vi "SPCM_simple_measure.vi"(2 "Clear memory":bool=TRUE, 3 "Collection Time":sgl=3.0 format="%.4f", 4 "Meas page":u16) -> (0 "SPC error":T3={"Error code"=0, "Message"="No errors"}, 1 "Waveform Graph":u16[][](graph))   [LabVIEW 2011]
uses:
  Program Files (x86)/BH/SPCM/DLL/spcm_functions_lv10.llb/error.ctl
  Program Files (x86)/BH/SPCM/DLL/spcm_functions_lv10.llb/Global_SPCM_vars.vi
  SPCM_DLL_path.vi
panel:
  in  "Active module":u16(ring) items=["Module 0", "Module 1", "Module 2", "Module 3", "Module 4", "Module 5", "Module 6", "Module 7"]
  out "Modules in use":T1
  in  "No of routing bits":u16 max=14 step=1
  in  "ADC resolution":u16=10 min=6 max=12 step=2
  out "SPC_rates":T2 {"Adc_rate" format="%.2e"; "Tac_rate" format="%.2e"; "Cfd_rate" format="%.2e"; "Sync_rate" format="%.2e"}
  in  "Current Collection Time":sgl=3.0 format="%.4f"
  in  "Current page":u16
  out "Output Array":u16[][](array[numeric])
  in  "Repeat Measurement":bool
  out "SYNC LED":bool=TRUE
  out "state value":i16 format="%.0x"
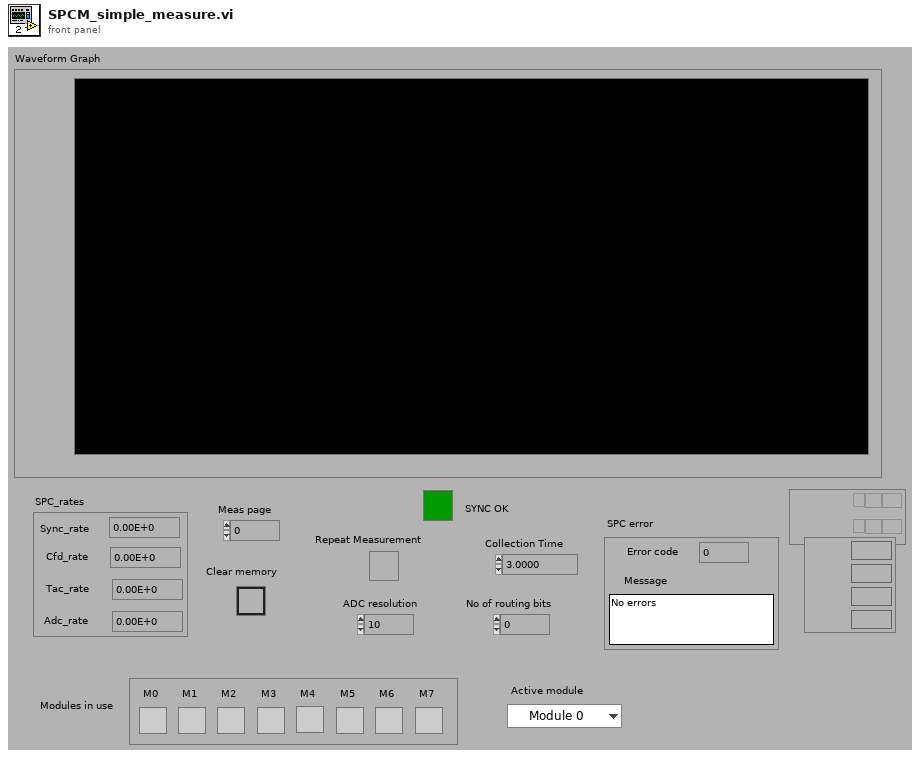
[diagram p1: front panel]
types:
  T1 = cluster{"M0":bool, "M1":bool, "M2":bool, "M3":bool, "M4":bool, "M5":bool, "M6":bool, "M7":bool}
  T2 = cluster{"Sync_rate":sgl, "Cfd_rate":sgl, "Tac_rate":sgl, "Adc_rate":sgl}
  T3 = typedef "error.ctl" = cluster{"Error code":i16, "Message":string}
  T4 = typedef "SPCdata.ctl" = cluster{"Base Address":u16, "Init status":i16, "CFD Limit Low [mV]":sgl, "CFD Limit High [mV]":sgl, "CFD ZC Level [mV]":sgl, "CFD Holdoff [ns]":sgl, "SYNC ZC Level [mV]":sgl, "SYNC Holdoff [ns]":sgl, "SYNC Threshold [mV]":sgl, "TAC Range [ns]":sgl, "SYNC Freq Divider":i16, "TAC Gain":i16, "TAC Offset [%]":sgl, "TAC Limit Low [%]":sgl, "TAC Limit High [%]":sgl, "ADC Resolution":i16, "Ext Latch Delay":i16, "Collection Time [s]":sgl, "Display Time [s]":sgl, "Repeat Time [s]":sgl, "Stop on Time":i16, "Stop on Overflow":i16, "Dither Range":i16, "Count Increment":i16, "Memory Bank":i16, "Dead Time Compensation":i16, "Scan Control":u16, "Routing Mode":i16, "TAC Enable Hold":sgl, "Slot No of PCI Module":i16, "Operation Mode":u16, "Scan Size X":u32, "Scan Size Y":u32, "Scan Routing Size X ":u32, "Scan Routing Size Y":u32, "Scan Flyback":u32, "Scan Borders":u32, "Scan Polarity":u16, "Pixel Clock Source":u16, "Line Compression":u16, "External Trigger Condition":u16, "Pixel Time [s]":sgl, "External pixel clock divider":u32, "Rate Counting Time":sgl, "Macro Time Clock  ":i16, "ADD Signal Source":i16, "Test EEPROM":i16, "ADC Zoom":i16, "Image Size X":u32, "Image Size Y":u32, "Image Routing Size X":u32, "Image Routing Size Y":u32, "XY Gain":i16, "Master Clock":i16, "ADC Sample Delay":i16, "Detector Type":i16, "X Axis Type":i16, "Channel enable ( DPC-230)":u32, "Channel slope ( DPC-230)":u32, "Channel spec_no ( DPC-230)":u32}
  T5 = typedef "mem_config.ctl" = cluster{"max_block_no":i32, "blocks_per_frame":i32, "frames_per_page":i32, "maxpage":i32, "block_length":i16}
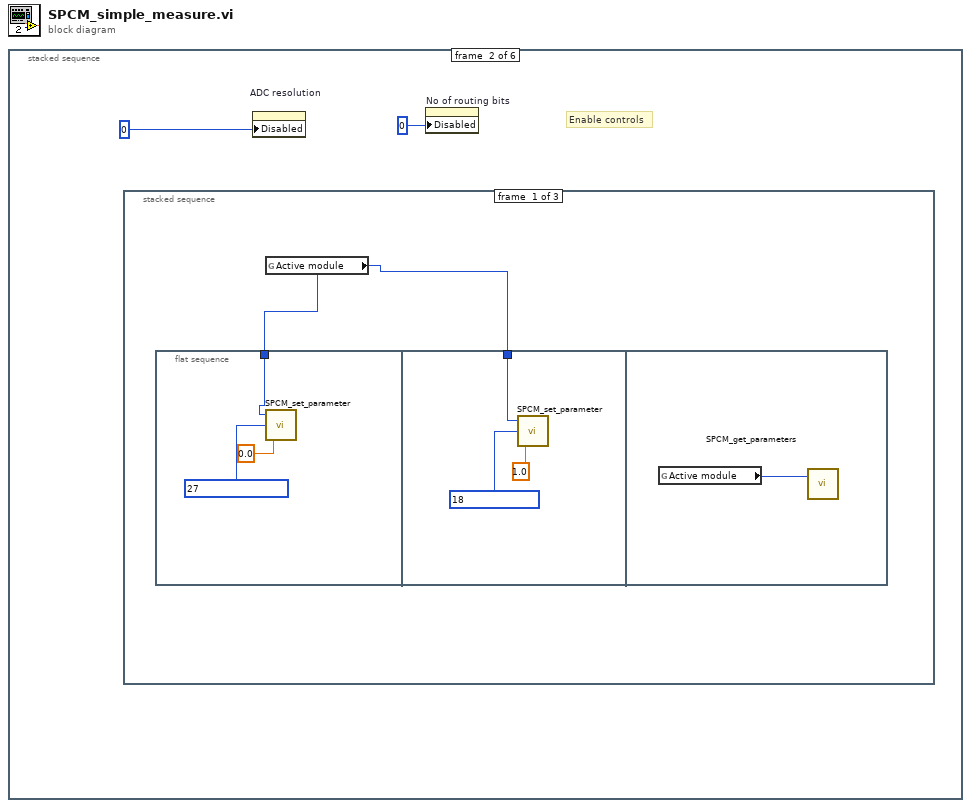
[diagram p0: block diagram]
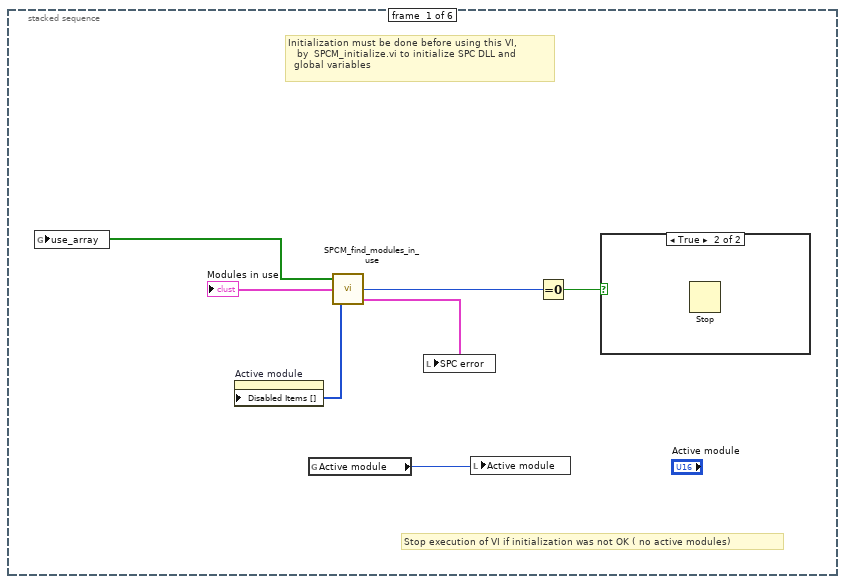
[diagram p2: hidden frame]
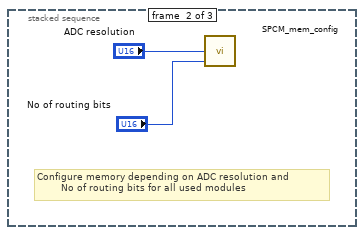
[diagram p4: hidden frame]
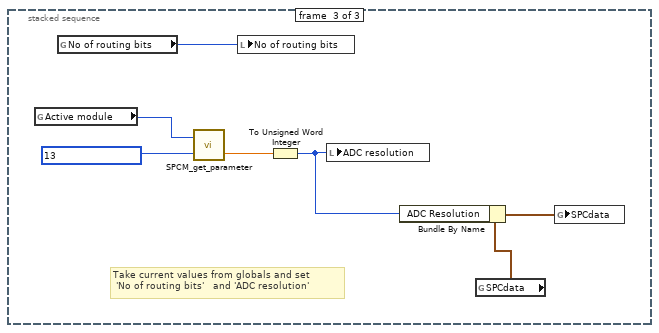
[diagram p5: hidden frame]
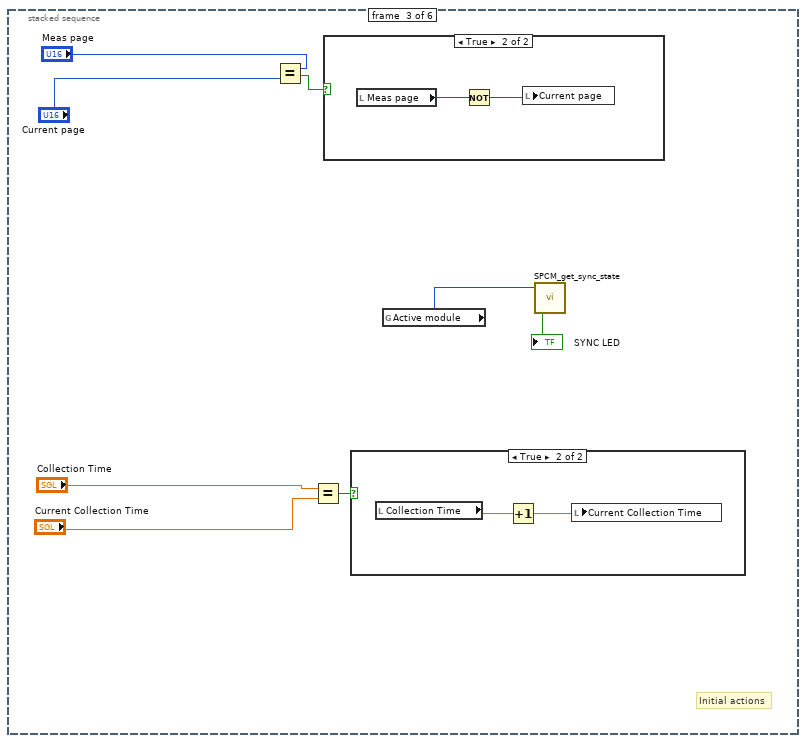
[diagram p6: hidden frame]
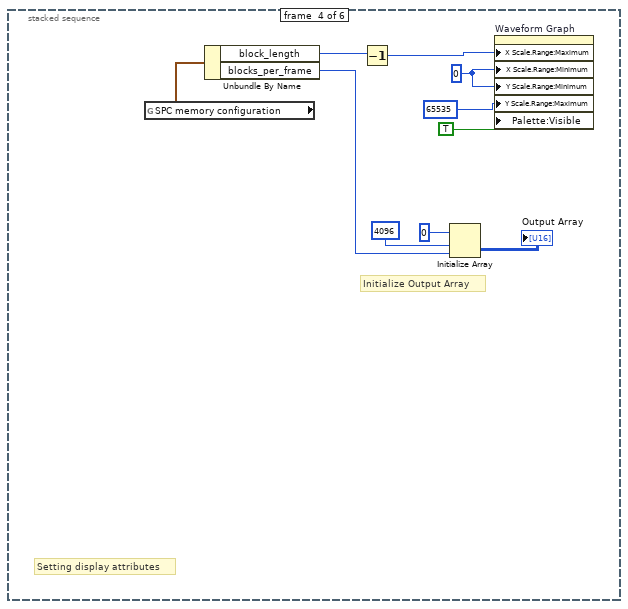
[diagram p9: hidden frame]
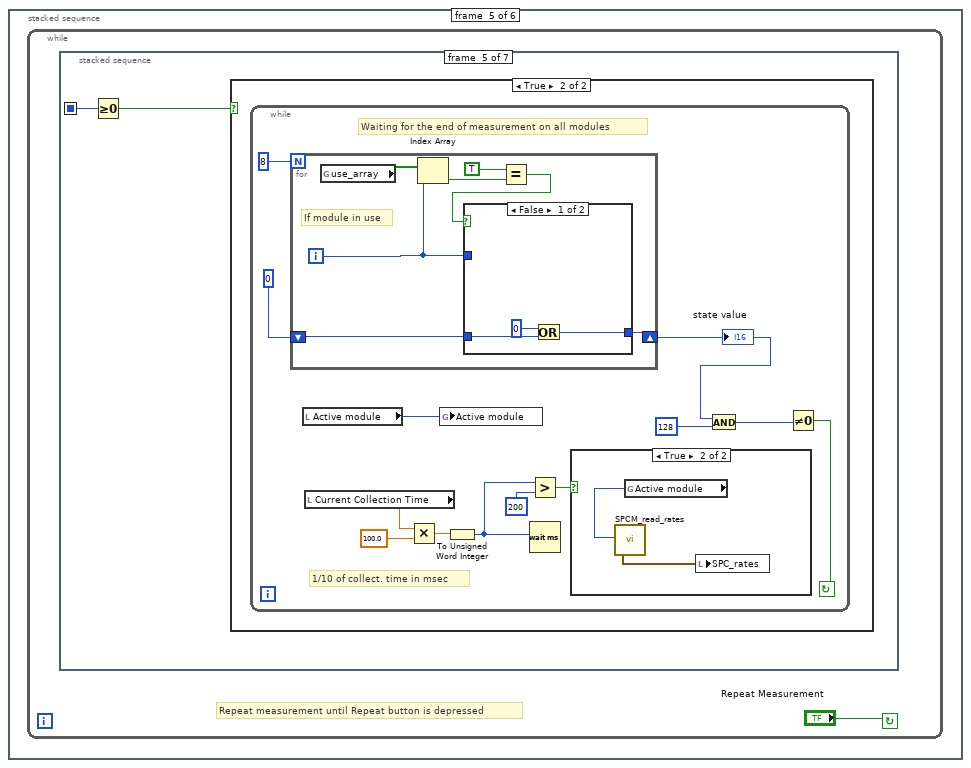
[diagram p10: hidden frame]
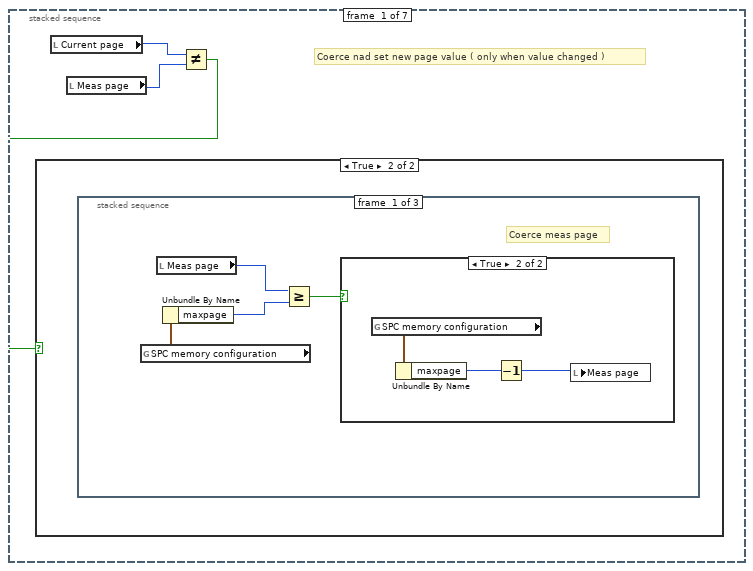
[diagram p11: hidden frame]
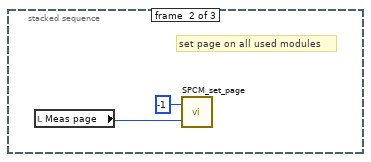
[diagram p14: hidden frame]
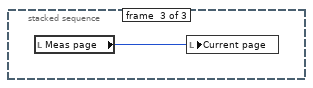
[diagram p15: hidden frame]
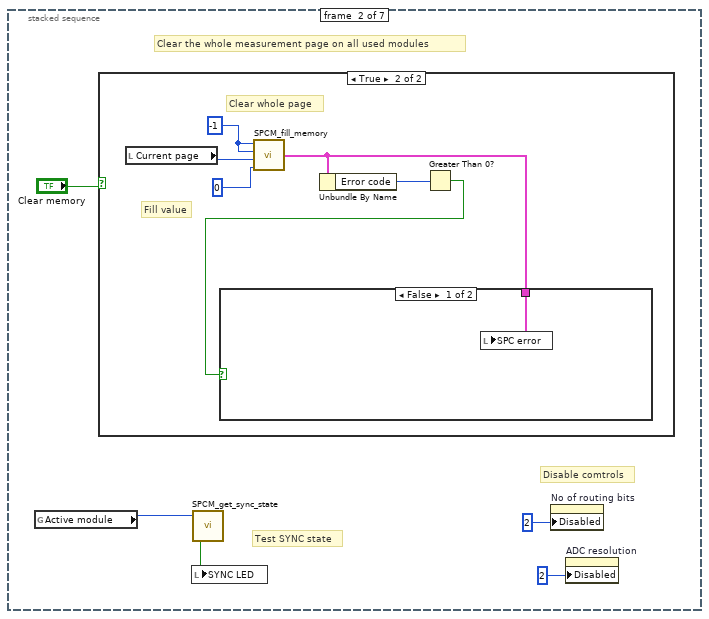
[diagram p16: hidden frame]
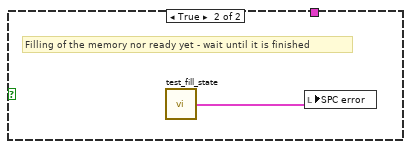
[diagram p18: hidden frame]
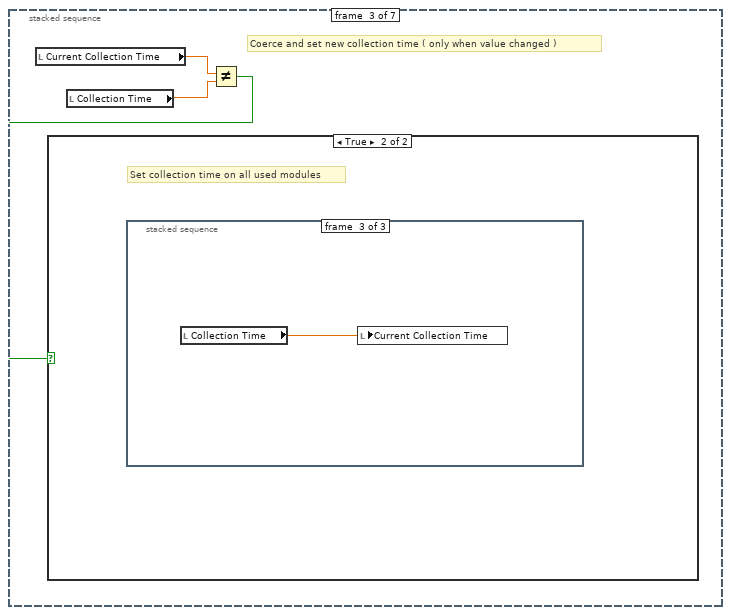
[diagram p19: hidden frame]
diagram:
  n1 = stacked-sequence {
    frame #0 {
      # "Stop execution of VI if initialization was not OK ( no active modules)"
      # "Initialization must be done before using this VI, \n   by  SPCM_initialize.vi to initialize SPC DLL and \n  global variables"
      n2 = global read "Global_SPCM_vars.vi" "Active module"() -> (w2:i16)
      n3 = call "SPCM_find_modules_in_use.vi"() -> ("SPC error"=w6:T3, "Number of used modules"=w4:i16, "Disabled Items"=w3:i32[], "Use LEDs"=→"Modules in use":T1, "use_array"=w1:bool[])  [unwired: 1 out]
      n4 = global write "Global_SPCM_vars.vi" "use_array"(w1) -> ()
      n5 = property on="Active module" class="Ring (strict)"("Disabled Items []"=w3) -> ()  [unwired: 2 in, 2 out]
      n6 = local write "SPC error"(w6) -> ()
      n7 = local write "Active module"(w2) -> ()
      n8 = Equal To 0?(x=w4) -> (x = 0?=w5:bool)
      n9 = case shown="True" w5 {
        frame False {
        }
        frame True {
          n10 = Stop() -> ()  [unwired: 1 in]
        }
      }
    }
    frame #1 {
      # "Enable controls"
      n11 = stacked-sequence {
        frame #0 {
          n12 = flat-sequence {
            tunnel: w10 -> [w11]
            tunnel: w10 -> [w14]
            frame #0 {
              n13 = call "SPCM_set_parameter.vi"("Parameter Value"=sgl 0.0, "SPC parameter ID"=u16 27, "Module no"=w11) -> ()  [unwired: 1 out]
            }
            frame #1 {
              n14 = call "SPCM_set_parameter.vi"("Parameter Value"=sgl 1.0, "SPC parameter ID"=u16 18, "Module no"=w14) -> ()  [unwired: 1 out]
            }
            frame #2 {
              n15 = global read "Global_SPCM_vars.vi" "Active module"() -> (w17:i16)
              n16 = call "SPCM_get_parameters.vi"("Module no"=w17) -> ()  [unwired: 2 out]
            }
          }
          n17 = global read "Global_SPCM_vars.vi" "Active module"() -> (w10:i16)
        }
        frame #1 {
          # "Configure memory depending on ADC resolution and\n        No of routing bits for all used modules"
          n18 = call "SPCM_mem_config.vi"("No of routing bits"="No of routing bits", "ADC resolution"="ADC resolution") -> ()  [unwired: 1 in, 2 out]
        }
        frame #2 {
          # "Take current values from globals and set\n 'No of routing bits'   and 'ADC resolution'"
          n19 = global read "Global_SPCM_vars.vi" "Active module"() -> (w23:i16)
          n20 = global read "Global_SPCM_vars.vi" "No of routing bits"() -> (w24:u16)
          n21 = call "SPCM_get_parameter.vi"("SPC parameter ID"=u16 13, "Module no"=w23) -> ("Current Parameter Value"=w26:sgl)  [unwired: 1 out]
          n22 = local write "No of routing bits"(w24) -> ()
          n23 = To Unsigned Word Integer(number=w26) -> (unsigned 16bit integer=w25:u16)
          n24 = local write "ADC resolution"(w25) -> ()
          n25 = global read "Global_SPCM_vars.vi" "SPCdata"() -> (w21:T4)
          n26 = Bundle By Name(cluster=w21, "ADC Resolution"=w25) -> (w22:T4)
          n27 = global write "Global_SPCM_vars.vi" "SPCdata"(w22) -> ()
        }
      }
      n28 = property on="ADC resolution" class="DigNum (strict)"("Disabled"=u8 0 ("Write Attribute")) -> ()  [unwired: 2 in, 2 out]
      n29 = property on="No of routing bits" class="DigNum (strict)"("Disabled"=u8 0 ("Write Attribute")) -> ()  [unwired: 2 in, 2 out]
    }
    frame #2 {
      # "Initial actions"
      n30 = Equal?(x="Meas page", y="Current page") -> (x = y?=w31:bool)
      n31 = Equal?(x="Collection Time", y="Current Collection Time") -> (x = y?=w28:bool)
      n32 = case shown="True" w31 {
        frame False {
        }
        frame True {
          n33 = local read "Meas page"() -> (w38:u16)
          n34 = Not(x=w38) -> (.not. x?=w37:u16)
          n35 = local write "Current page"(w37) -> ()
        }
      }
      n36 = case shown="True" w28 {
        frame False {
        }
        frame True {
          n37 = local read "Collection Time"() -> (w36:sgl)
          n38 = Increment(x=w36) -> (x+1=w35:sgl)
          n39 = local write "Current Collection Time"(w35) -> ()
        }
      }
      n40 = global read "Global_SPCM_vars.vi" "Active module"() -> (w27:i16)
      n41 = call "SPCM_get_sync_state.vi"("Module no"=w27) -> ("LED"=→"SYNC LED":bool)  [unwired: 2 out]
    }
    frame #3 {
      w43 = u16 0 ("Write Attribute")
      # "Initialize Output Array"
      # "Setting display attributes"
      n42 = global read "Global_SPCM_vars.vi" "SPC memory configuration"() -> (w48:T5)
      n43 = Unbundle By Name(w48) -> ("block_length"=w40:i16, "blocks_per_frame"=w44:i32)
      n44 = Decrement(x=w40) -> (x-1=w47:i16)
      n45 = Initialize Array(u16 0 ("Element Data"), 4096 ("Dimension Size"), w44) -> (→"Output Array":u16[][])
      n46 = property on="Waveform Graph" class="WFGraph (strict)"("X Scale.Range:Maximum"=w47, "X Scale.Range:Minimum"=w43, "Y Scale.Range:Minimum"=w43, "Y Scale.Range:Maximum"=u16 65535 ("Write Attribute"), "Palette:Visible"=TRUE ("Write Attribute")) -> ()  [unwired: 2 in, 2 out]
    }
    frame #4 {
      n47 = while {
        stop <- "Repeat Measurement" continue-if-true
        # "Repeat measurement until Repeat button is depressed"
        n48 = stacked-sequence {
          seq-local: [_ _ _ w88 _ _ _] -> [_ _ _ _ w104 w135 _]
          frame #0 {
            # "Coerce nad set new page value ( only when value changed )"
            n49 = local read "Current page"() -> (w52:u16)
            n50 = local read "Meas page"() -> (w50:u16)
            n51 = Not Equal?(x=w52, y=w50) -> (x != y?=w51:bool)
            n52 = case shown="True" w51 {
              frame False {
              }
              frame True {
                n53 = stacked-sequence {
                  frame #0 {
                    # "Coerce meas page"
                    n54 = global read "Global_SPCM_vars.vi" "SPC memory configuration"() -> (w56:T5)
                    n55 = local read "Meas page"() -> (w53:u16)
                    n56 = Unbundle By Name(w56) -> ("maxpage"=w55:i32)
                    n57 = Greater Or Equal?(x=w53, y=w55) -> (x >= y?=w54:bool)
                    n58 = case shown="True" w54 {
                      frame False {
                      }
                      frame True {
                        n59 = global read "Global_SPCM_vars.vi" "SPC memory configuration"() -> (w59:T5)
                        n60 = Unbundle By Name(w59) -> ("maxpage"=w58:i32)
                        n61 = Decrement(x=w58) -> (x-1=w57:i32)
                        n62 = local write "Meas page"(w57) -> ()
                      }
                    }
                  }
                  frame #1 {
                    # "set page on all used modules"
                    n63 = local read "Meas page"() -> (w61:u16)
                    n64 = call "SPCM_set_page.vi"("Page"=w61, "Module no"=i16 -1) -> ()  [unwired: 1 out]
                  }
                  frame #2 {
                    n65 = local read "Meas page"() -> (w62:u16)
                    n66 = local write "Current page"(w62) -> ()
                  }
                }
              }
            }
          }
          frame #1 {
            # "Disable comtrols"
            # "Test SYNC state"
            # "Clear the whole measurement page on all used modules"
            n67 = global read "Global_SPCM_vars.vi" "Active module"() -> (w65:i16)
            n68 = case shown="True" "Clear memory" {
              frame False {
              }
              frame True {
                w71 = i16 -1 ("Block")
                # "Clear whole page"
                # "Fill value"
                n69 = local read "Current page"() -> (w72:u16)
                n70 = call "SPCM_fill_memory.vi"("Fill value"=u16 0, "Page"=w72, "Block"=w71, "Module no"=w71) -> ("SPC error"=w68:cluster{"Error code":i16, "Message":string})
                n71 = Unbundle By Name(w68) -> ("Error code"=w69:i16)
                n72 = Greater Than 0?(x=w69) -> (x > 0?=w70:bool)
                n73 = case shown="False" w70 {
                  tunnel: w68 -> [w74 _]
                  frame False {
                    n74 = local write "SPC error"(w74) -> ()
                  }
                  frame True {
                    # "Filling of the memory nor ready yet - wait until it is finished"
                    n75 = call "test_fill_state.vi"() -> ("SPC error"=w75:T3)  [unwired: 1 out]
                    n76 = local write "SPC error"(w75) -> ()
                  }
                }
              }
            }
            n77 = call "SPCM_get_sync_state.vi"("Module no"=w65) -> ("LED"=w66:bool)  [unwired: 2 out]
            n78 = local write "SYNC LED"(w66) -> ()
            n79 = property on="No of routing bits" class="DigNum (strict)"("Disabled"=u8 2 ("Write Attribute")) -> ()  [unwired: 2 in, 2 out]
            n80 = property on="ADC resolution" class="DigNum (strict)"("Disabled"=u8 2 ("Write Attribute")) -> ()  [unwired: 2 in, 2 out]
          }
          frame #2 {
            # "Coerce and set new collection time ( only when value changed )"
            n81 = local read "Current Collection Time"() -> (w78:sgl)
            n82 = local read "Collection Time"() -> (w77:sgl)
            n83 = Not Equal?(x=w78, y=w77) -> (x != y?=w76:bool)
            n84 = case shown="True" w76 {
              frame False {
              }
              frame True {
                # "Set collection time on all used modules"
                n85 = stacked-sequence {
                  frame #0 {
                    n86 = local read "Collection Time"() -> (w81:sgl)
                    n87 = call "SPCM_set_parameter.vi"("Parameter Value"=w81, "SPC parameter ID"=u16 15, "Module no"=i16 -1) -> ()  [unwired: 1 out]
                  }
                  frame #1 {
                    n88 = global read "Global_SPCM_vars.vi" "Active module"() -> (w83:i16)
                    n89 = call "SPCM_get_parameter.vi"("SPC parameter ID"=u16 15, "Module no"=w83) -> ("Current Parameter Value"=w86:sgl)  [unwired: 1 out]
                    n90 = local write "Collection Time"(w86) -> ()
                    n91 = global read "Global_SPCM_vars.vi" "SPCdata"() -> (w84:T4)
                    n92 = Bundle By Name(cluster=w84, "Collection Time [s]"=w86) -> (w85:T4)
                    n93 = global write "Global_SPCM_vars.vi" "SPCdata"(w85) -> ()
                  }
                  frame #2 {
                    n94 = local read "Collection Time"() -> (w87:sgl)
                    n95 = local write "Current Collection Time"(w87) -> ()
                  }
                }
              }
            }
          }
          frame #3 {
            # "Start measurement on all used modules"
            n96 = for {
              N: 8 -> [_]
              shift-right: [w92] -> w88
              shift-left: 0 -> [w93]
              i -> [w94]
              # "If module in use"
              n97 = global read "Global_SPCM_vars.vi" "use_array"() -> (w91:bool[])
              n98 = Index Array(array=w91, index=w94) -> (element=w97:bool)
              n99 = Equal?(x=TRUE, y=w97) -> (x = y?=w95:bool)
              n100 = case shown="True" w95 {
                tunnel: w94 -> [_ w103]
                tunnel: w93 -> [w98 w101]
                tunnel: [w98 w99] -> w92
                frame False {
                }
                frame True {
                  n101 = call "SPCM_start_meas.vi"("Module no"=w103) -> ("SPC error"=w102:cluster{"Error code":i16, "Message":string})
                  "SPC error" <- w102
                  n102 = Unbundle By Name(w102) -> ("Error code"=w100:i16)
                  n103 = Or(x=w100, y=w101) -> (x .or. y?=w99:i32)
                }
              }
            }
          }
          frame #4 {
            n104 = Greater Or Equal To 0?(x=w104) -> (x >= 0?=w105:bool)
            n105 = case shown="True" w105 {
              frame False {
              }
              frame True {
                n106 = while {
                  stop <- w116 continue-if-true
                  # "Waiting for the end of measurement on all modules"
                  # "1/10 of collect. time in msec"
                  n107 = for {
                    N: 8 -> [_]
                    shift-right: [w124] -> w106
                    shift-left: 0 -> [w125]
                    i -> [w120]
                    # "If module in use"
                    # "Test if still Armed"
                    n108 = global read "Global_SPCM_vars.vi" "use_array"() -> (w121:bool[])
                    n109 = Index Array(array=w121, index=w120) -> (element=w123:bool)
                    n110 = Equal?(x=TRUE, y=w123) -> (x = y?=w119:bool)
                    n111 = case shown="False" w119 {
                      tunnel: w125 -> [w128 w131]
                      tunnel: [w127 w130] -> w124
                      tunnel: w120 -> [_ w129]
                      frame False {
                        n112 = Or(x=0, y=w128) -> (x .or. y?=w127:i32)
                      }
                      frame True {
                        n113 = call "SPCM_test_state.vi"("Module no"=w129) -> ("state value"=w132:i16)  [unwired: 1 out]
                        n114 = Or(x=w132, y=w131) -> (x .or. y?=w130:i32)
                      }
                    }
                  }
                  "state value" <- w106
                  n115 = local read "Active module"() -> (w107:u16)
                  n116 = local read "Current Collection Time"() -> (w111:sgl)
                  n117 = Multiply(x=w111, y=sgl 100.0) -> (x*y=w114:sgl)
                  n118 = global write "Global_SPCM_vars.vi" "Active module"(w107) -> ()
                  n119 = To Unsigned Word Integer(number=w114) -> (unsigned 16bit integer=w110:u16)
                  n120 = Greater?(x=w110, y=u16 200) -> (0:w113:bool)
                  n121 = Wait (ms)(milliseconds to wait=w110) -> ()  [unwired: 1 out]
                  n122 = case shown="True" w113 {
                    frame False {
                    }
                    frame True {
                      n123 = global read "Global_SPCM_vars.vi" "Active module"() -> (w133:i16)
                      n124 = call "SPCM_read_rates.vi"("Module no"=w133) -> ("SPC_rates"=w134:T2)  [unwired: 1 out]
                      n125 = local write "SPC_rates"(w134) -> ()
                    }
                  }
                  n126 = And(x=w106, y=u16 128) -> (x .and. y?=w117:i32)
                  n127 = Not Equal To 0?(x=w117) -> (x != 0?=w116:bool)
                }
              }
            }
          }
          frame #5 {
            n128 = Greater Or Equal To 0?(x=w135) -> (x >= 0?=w136:bool)
            n129 = case shown="True" w136 {
              frame False {
              }
              frame True {
                # "reading all blocks from\n    the actual page"
                n130 = global read "Global_SPCM_vars.vi" "SPC memory configuration"() -> (w138:T5)
                n131 = Unbundle By Name(w138) -> ("blocks_per_frame"=w137:i32)
                n132 = for {
                  N: w137 -> [_]
                  i -> [w141]
                  # "Exchange one column\nin Output Array with data\nfrom Data Array"
                  # "Block"
                  # "Reduction"
                  # "To"
                  # "From"
                  # "reading results"
                  n133 = global read "Global_SPCM_vars.vi" "SPC memory configuration"() -> (w153:T5)
                  n134 = Unbundle By Name(w153) -> ("block_length"=w150:i16)
                  n135 = global read "Global_SPCM_vars.vi" "Active module"() -> (w140:i16)
                  n136 = local read "Current page"() -> (w142:u16)
                  n137 = global read "SPCM_DLL_path.vi" "DLL_path"() -> (w139:path)
                  n138 = Decrement(x=w150) -> (x-1=w145:i16)
                  n139 = global read "Global_SPCM_vars.vi" "MData Array"() -> (w147:u16[])
                  n140 = local read "Output Array"() -> (w149:u16[][])
                  n141 = dll-call lib="D:/spcm/lib/lab_view/lv10.0/spcm32.dll" fn="SPC_read_data_block"(path in=w139, "mod_no"=w140, "block"=w141, "page"=w142, "reduction_factor"=i16 1, "from"=i16 0 ("From"), "to"=w145, "data"=w147) -> ("return type"=w152:i16, "data"=w146:u16[])  [unwired: 8 in, 2 out]
                  n142 = global write "Global_SPCM_vars.vi" "MData Array"(w146) -> ()
                  n143 = call "SPCM_get_error_string.vi"("Error code"=w152) -> ("SPC error"=w151:cluster{"Error code":i16, "Message":string})
                  n144 = for {
                    shift-right: [w157] -> w148
                    shift-left: w149 -> [w158]
                    tunnel: w141 -> [w155]
                    tunnel: w146 -> [w154] mode=indexing
                    tunnel: [w154] -> _ mode=indexing
                    i -> [w156]
                    n145 = Replace Array Subset(array=w158, new element=w154, index (row)=w156, index (col)=w155) -> (w157:u16[][])
                  }
                  n146 = local write "Output Array"(w148) -> ()
                  n147 = local write "SPC error"(w151) -> ()
                }
              }
            }
          }
          frame #6 {
            # "Save one block to spc_test.sdt file"
            # "Display results\n(all blocks from the current page)"
            n148 = stacked-sequence {
              tunnel: [w167] -> w166
              frame #0 {
                n149 = local read "Active module"() -> (w167:u16)
                n150 = global write "Global_SPCM_vars.vi" "Active module"(w167) -> ()
              }
            }
            n151 = stacked-sequence {
              tunnel: w166 -> [w168]
              frame #0 {
                # "Read Rates"
                n152 = call "SPCM_read_rates.vi"("Module no"=w168) -> ("SPC_rates"=→"SPC_rates":T2)  [unwired: 1 out]
              }
            }
            n153 = local read "Output Array"() -> (→"Waveform Graph":u16[][])
            n154 = global read "Global_SPCM_vars.vi" "MData Array"() -> (w159:u16[])
            n155 = global read "Global_SPCM_vars.vi" "SPC memory configuration"() -> (w164:T5)
            n156 = Unbundle By Name(w164) -> ("block_length"=w162:i16)
            n157 = Multiply(x=w162, y=i16 2) -> (x*y=w161:i16)
            n158 = call "SPCM_save_data_to_sdtfile.vi"("No of bytes to save"=w161, "data_buf"=w159, "Module no"=w166) -> ("SPC error"=w165:cluster{"Error code":i16, "Message":string})  [unwired: 1 in]
            n159 = local write "SPC error"(w165) -> ()
          }
        }
      }
    }
    frame #5 {
      n160 = global read "Global_SPCM_vars.vi" "Active module"() -> (w170:i16)
      n161 = property on="No of routing bits" class="DigNum (strict)"("Disabled"=u8 0 ("Write Attribute")) -> ()  [unwired: 2 in, 2 out]
      n162 = property on="ADC resolution" class="DigNum (strict)"("Disabled"=u8 0 ("Write Attribute")) -> ()  [unwired: 2 in, 2 out]
      n163 = call "SPCM_get_parameters.vi"("Module no"=w170) -> ()  [unwired: 2 out]
    }
  }
